vi "F8588A Digitizing Process.vi"(8 "error in":errorcluster, 11 "session in":variant) -> (0 "error out":errorcluster, 3 "aux data out":variant)   [LabVIEW 2020]
doc: "3458A digitizing lib: Main digitizing process. The VI is assynchronously executed once for each channel (all in parallel). It is started by calling 'Initiate Digitizing Process'. It then samples and sends the digitized data via queues to main process where the data are collected using 'Fetch Digitized Data'. Configuration of the execution is stored in 'session in' variable, execution control details are in 'session in->proc setup' cluster. Each instance of this VI has ID starting from 0 which identifies to which channel it belongs to."
uses:
  DMM/3458A Digitizer Session.ctl
  DMM/3458A Virtual Channel Config.ctl
  Counter/Counter Session.ctl
  Counter/Counter Type.ctl
  AWG/AWG Session.ctl
  AWG/AWG Type.ctl
  AWG/CMI Clock Divider v2/CMI ckd2 Session.ctl
  AWG/CMI Clock Divider v2/CMI ckd2 Source Mode.ctl
  AWG/CMI Sync V3/CMI Sync V3 session.ctl
  AWG/CMI Sync V3/Configure/CMI Sync V3 Reference Clock Source.ctl
  AWG/CMI Sync V3/Configure/CMI Sync V3 HV input Range.ctl
  AWG/CMI Sync V3/Configure/CMI Sync V3 Trigger Input Level.ctl
  AWG/CMI Sync V3/Configure/CMI Sync V3 Channel 1 Mode.ctl
  AWG/CMI Sync V3/Configure/CMI Sync V3 Channel Output Levels.ctl
  AWG/CMI Sync V3/Configure/CMI Sync V3 Channel 2 Mode.ctl
  AWG/CMI Sync V3/Configure/CMI Sync V3 Channel 3 Mode.ctl
  DMM/3458A Sync Mode.ctl
  DMM/3458A Idn Mode.ctl
  DMM/3458A Digitizing Low Levels/Configure/Sampling Mode.ctl
  DMM/3458A Digitizing Process Options.ctl
  DMM/3458A Data Packet.ctl
  DMM/3458A Aux Record Data.ctl
  DMM/3458A Digitizing Low Levels/Configure/Level Setup.ctl
  DMM/3458A Digitizing Low Levels/Configure/First Sample Trigger.ctl
  DMM/3458A Aperture Selection Mode.ctl
  DMM/3458A Multiplexing Config.ctl
  F8588A Low Pass Filter.ctl
  F8588A Phase Lock.ctl
  F8588A Coupling.ctl
  <vilib>/Utility/error.llb/Error Cluster From Error Code.vi
  <vilib>/ErrorRing/Error Ring.xnode
  DMM/3458A Virtual Digitizer.lvlib
  Counter/Counter.lvlib
  AWG/AWG.lvlib
  DMM/3458A Digitizing Low Levels/3458A Digitizing Low Levels.lvlib
  AWG/CMI Sync V3/CMI Sync Unit V3.lvlib
  AWG/AWG Clock Setup Mode.ctl
  DMM/3458A Sampling Rate.ctl
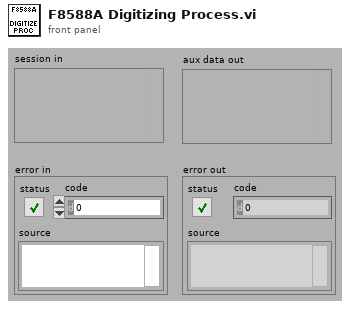
[diagram p1: front panel]
types:
  T1 = typedef "3458A Virtual Digitizer.lvlib/3458A Data Packet.ctl" = cluster{"data":i32[][], "offset [smpl]":i32, "count [smpl]":i32, "all done?":bool, "sampling?":bool, "queue buffer [%]":dbl, "valid?":bool, "overflow?":bool}
  T2 = typedef "3458A Virtual Digitizer.lvlib/3458A Digitizer Session.ctl" = cluster{"channels":T3[], "sync unit":T4, "awg unit":T6, "sync mode":T18, "streaming mode":bool, "idn mode":T19, "sampling mode":T20, "sample memory [B]":i32, "proc setup":T21, "sample size [B]":i32, "sample count":i32, "aux data":T23, "ranges [V]":dbl[], "aperture [s]":dbl, "LEVEL trigger":T24, "trigger mode":T25, "measure temp.?":bool, "disp mesages":string[], "shared bus?":bool, "disable display?":bool, "aper mode":T26, "aper rules":dbl[][], "multiplex":T27, "F8588 lpf":T28, "F8588 pll":T29, "F8588 couple":T30, "fs":T31}
  T3 = typedef "3458A Virtual Digitizer.lvlib/3458A Virtual Channel Config.ctl" = cluster{"VISA":refnum<visa-resource-name>, "Range [Vpk]":dbl, "btn clr":bool, "btn up":bool, "btn down":bool, "F8588":bool, "F8588 guard":bool}
  T4 = typedef "Counter.lvlib/Counter Session.ctl" = cluster{"VISA":refnum<visa-resource-name>, "type":T5}
  T5 = typedef "Counter.lvlib/Counter Type.ctl" = enum16{"Picotest U6200A", "dummy"}
  T6 = typedef "AWG.lvlib/AWG Session.ctl" = cluster{"type":T7, "VISA":refnum<visa-resource-name>, "enable 10MHz ref":bool, "cmi ckd2":T8, "cmi sync v3":T10}
  T7 = typedef "AWG.lvlib/AWG Type.ctl" = enum16{"Agilent 331xxA to 332xxA", "Agilent 335xxA to 336xxA", "Tektronix AFG3101C", "CMI Clock Divider v2", "CMI Sync Unit V3", "dummy"}
  T8 = typedef "AWG.lvlib/CMI ckd2 Session.ctl" = cluster{"VISA":refnum<visa-resource-name>, "clock source":T9, "manual ref clk":bool, "ref clock [Hz]":dbl}
  T9 = typedef "AWG.lvlib/CMI ckd2 Source Mode.ctl" = enum16{"Auto", "LF clock", "HF clock", "Internal"}
  T10 = typedef "AWG.lvlib/CMI Sync Unit V3.lvlib/CMI Sync V3 session.ctl" = cluster{"VISA":refnum<visa-resource-name>, "baud rate [bd/s]":i32, "source":T11, "hv range":T12, "fsrc is fixed":bool, "fsrc [Hz]":dbl, "freq integ [s]":dbl, "freq filter":i32, "trig level":T13, "chn1 mode":T14, "chn1 level":T15, "chn2 mode":T16, "chn2 level":T15, "chn2 div":i32, "chn3 mode":T17, "chn3 level":T15}
  T11 = typedef "AWG.lvlib/CMI Sync Unit V3.lvlib/CMI Sync V3 Reference Clock Source.ctl" = enum16{"Auto", "Internal", "Logic", "Sine", "HV"}
  T12 = typedef "AWG.lvlib/CMI Sync Unit V3.lvlib/CMI Sync V3 HV input Range.ctl" = enum16{"10V", "60V", "250V", "1kV"}
  T13 = typedef "AWG.lvlib/CMI Sync Unit V3.lvlib/CMI Sync V3 Trigger Input Level.ctl" = enum16{"LVCMOS 3V3", "TTL 5V"}
  T14 = typedef "AWG.lvlib/CMI Sync Unit V3.lvlib/CMI Sync V3 Channel 1 Mode.ctl" = enum16{"Source divider", "DDS absolute", "DDS ratio", "DDS ratio M/N"}
  T15 = typedef "AWG.lvlib/CMI Sync Unit V3.lvlib/CMI Sync V3 Channel Output Levels.ctl" = enum16{"Positive 3V3", "Negative 3V3", "Positive 5V", "Negative 5V"}
  T16 = typedef "AWG.lvlib/CMI Sync Unit V3.lvlib/CMI Sync V3 Channel 2 Mode.ctl" = enum16{"Source divider", "Chn 1 divide"}
  T17 = typedef "AWG.lvlib/CMI Sync Unit V3.lvlib/CMI Sync V3 Channel 3 Mode.ctl" = enum16{"Chn 1 Active", "Chn 2 Active", "Chn 1 Trigger", "Chn 2 Trigger", "Gate", "PPS", "10MHz"}
  T18 = typedef "3458A Virtual Digitizer.lvlib/3458A Sync Mode.ctl" = enum16{"MASTER-SLAVE, MASTER clocked by TIMER", "MASTER-SLAVE, MASTER clocked by AWG", "ALL clocked by AWG", "MASTER-SLAVE, ALL clocked by TIMER", "ALL clocked by AWG with DFLL"}
  T19 = typedef "3458A Virtual Digitizer.lvlib/3458A Idn Mode.ctl" = enum16{"Auto", "Sequential (chn A, chn B, ...)", "From calibration string"}
  T20 = typedef "3458A Virtual Digitizer.lvlib/3458A Digitizing Low Levels.lvlib/Sampling Mode.ctl" = enum16{"DCV", "DSDC", "DSAC"}
  T21 = typedef "3458A Virtual Digitizer.lvlib/3458A Digitizing Process Options.ctl" = cluster{"channel id":i32, "packet size [smpl]":i32, "current timeout [s]":dbl, "blk2blk timeout [s]":dbl, "event time":timestamp, "stop notifier":refnum<notifier>, "data queues":refnum<queue>[], "proc refs":refnum<vi>[], "bus semaphore":T22}
  T22 = typedef "Semaphore RefNum" = refnum<k1>
  T23 = typedef "3458A Virtual Digitizer.lvlib/3458A Aux Record Data.ctl" = cluster{"channel id":i32, "valid?":bool[], "gain [V]":dbl[], "timestamp [s]":dbl[], "Ts [s]":dbl, "abs timestamp":timestamp, "t [deg C]":dbl[], "multiplex timestamp [s]":dbl, "only multiplex?":bool, "multiplex smpl offset":i64, "overflow?":bool}
  T24 = typedef "3458A Virtual Digitizer.lvlib/3458A Digitizing Low Levels.lvlib/Level Setup.ctl" = cluster{"edge":enum16{"POS", "NEG"}, "level [V]":dbl, "coupling":enum16{"DC", "AC"}}
  T25 = typedef "3458A Virtual Digitizer.lvlib/3458A Digitizing Low Levels.lvlib/First Sample Trigger.ctl" = enum16{"AUTO", "EXT", "SYN", "SGL", "HOLD", "LEVEL"}
  T26 = typedef "3458A Virtual Digitizer.lvlib/3458A Aperture Selection Mode.ctl" = enum16{"Manual", "Maximum", "Table"}
  T27 = typedef "3458A Multiplexing Config.ctl" = cluster{"cycles":i32, "delay [s]":dbl, "enabled":bool, "overhead [s]":dbl, "tot smpls":i64, "sub-rec":i32, "overhead [%]":dbl, "emulated":bool}
  T28 = typedef "F8588A Low Pass Filter.ctl" = enum16{"Off", "100 kHz", "3 MHz"}
  T29 = typedef "F8588A Phase Lock.ctl" = enum16{"Off", "1 MHz", "10 MHz"}
  T30 = typedef "F8588A Coupling.ctl" = enum16{"AC, 1 MOhm", "AC, 10 MOhm", "DC, 1 MOhm", "DC, 10 MOhm", "DC, auto"}
  T31 = typedef "3458A Virtual Digitizer.lvlib/3458A Sampling Rate.ctl" = cluster{"freq mode":T32, "fs [Hz]":dbl, "fref [Hz]":dbl, "mul":dbl, "div":dbl}
  T32 = typedef "AWG.lvlib/AWG Clock Setup Mode.ctl" = enum16{"fs or Ts", "fs or Ts with fref", "fref/N", "fref*M/N", "fref*Ratio"}
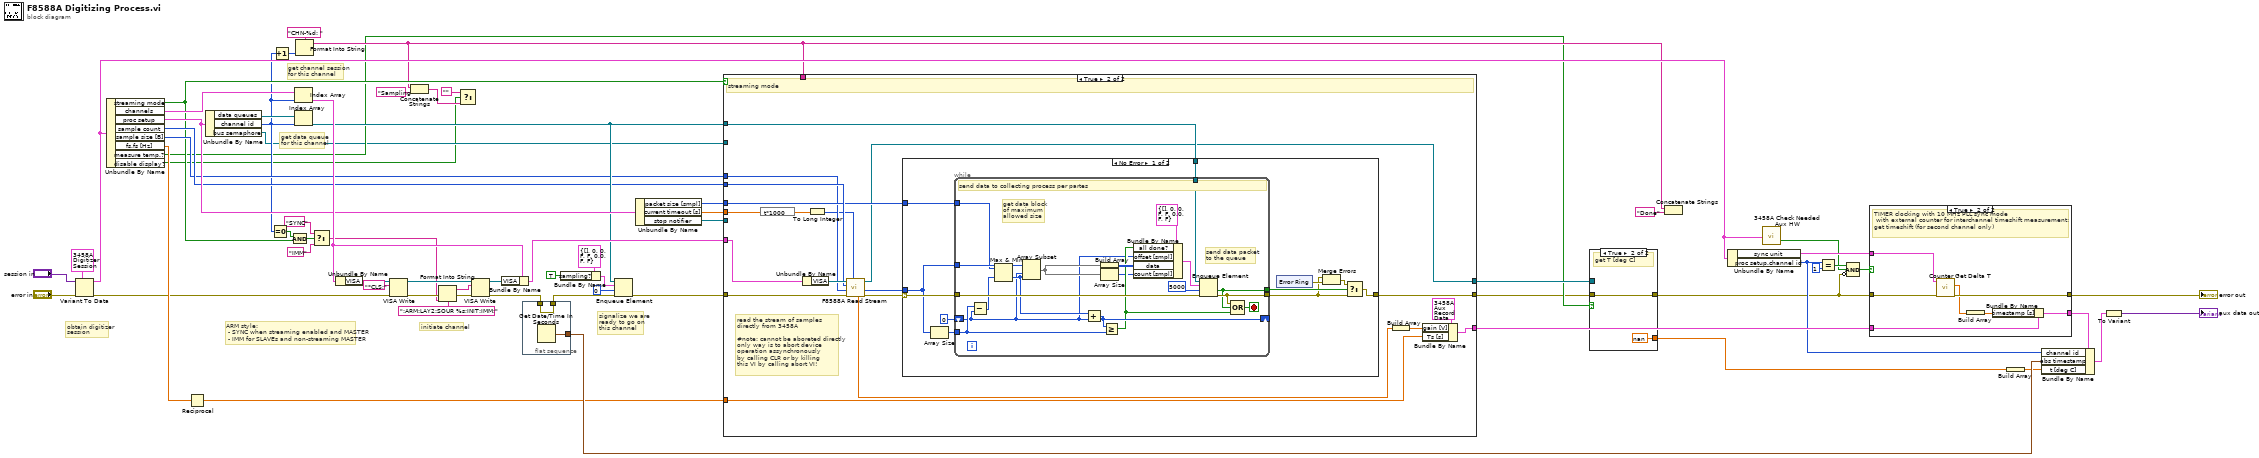
[diagram p0: block diagram]
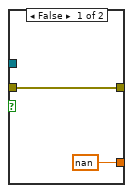
[diagram p2: hidden frame]
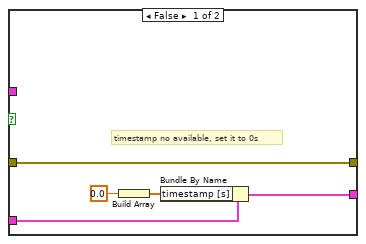
[diagram p3: hidden frame]
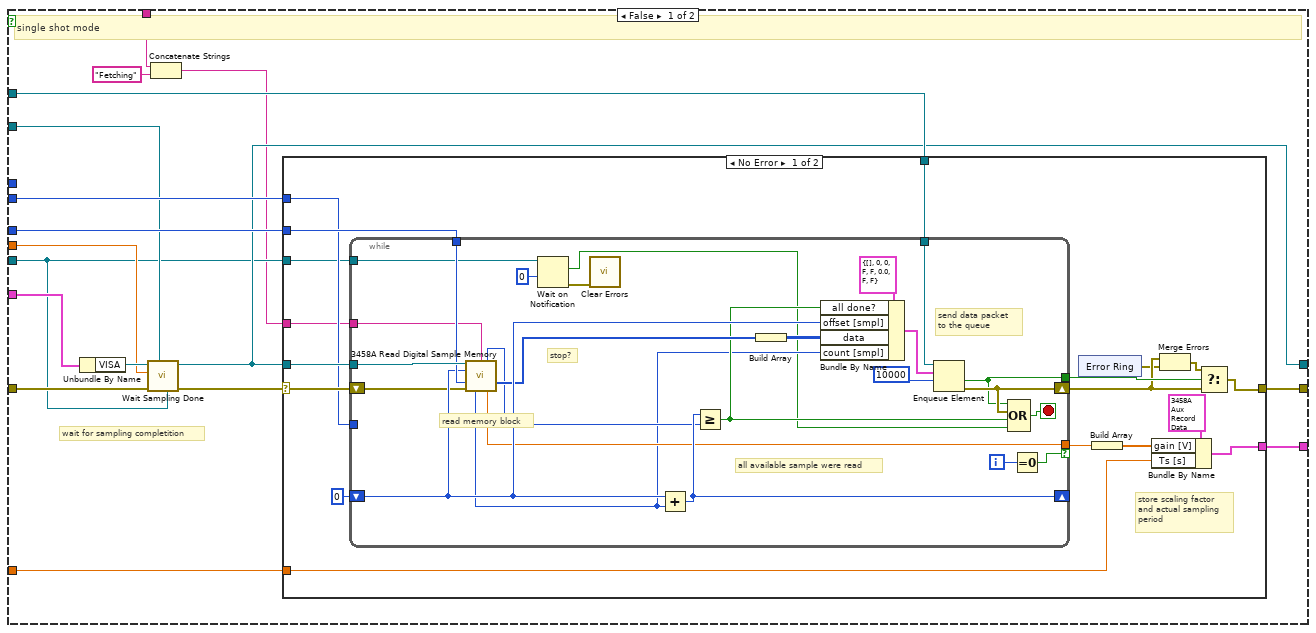
[diagram p4: hidden frame]
diagram:
  # "ARM style:\n - SYNC when streaming enabled and MASTER\n - IMM for SLAVEs and non-streaming MASTER"
  # "get channel session\nfor this channel"
  # "get data queue\nfor this channel"
  # "signalize we are\nready to go on \nthis channel"
  # "initiate channel"
  # "obtain digitizer\nsession"
  n1 = Variant To Data(error in="error in", type=T2 {"channels"=[], "sync unit"={"VISA"="", "type"=enum."Picotest U6200A"}, "awg unit"={"type"=enum."Agilent 331xxA to 332xxA", "VISA"="", "enable 10MHz ref"=FALSE, "cmi ckd2"={"VISA"="", "clock source"=enum."Auto", "manual ref clk"=FALSE, "ref clock [Hz]"=0.0}, "cmi sync v3"={"VISA"="", "baud rate [bd/s]"=115200, "source"=enum."Auto", "hv range"=enum."1kV", "fsrc is fixed"=FALSE, "fsrc [Hz]"=10000000.0, "freq integ [s]"=1.0, "freq filter"=5, "trig level"=enum."TTL 5V", "chn1 mode"=enum."Source divider", "chn1 level"=enum."Positive 5V", "chn2 mode"=enum."Source divider", "chn2 level"=enum."Positive 5V", "chn2 div"=1, "chn3 mode"=enum."Chn 1 Active", "chn3 level"=enum."Positive 5V"}}, "sync mode"=enum."MASTER-SLAVE, MASTER clocked by TIMER", "streaming mode"=FALSE, "idn mode"=enum."Auto", "sampling mode"=enum."DCV", "sample memory [B]"=0, "proc setup"={"channel id"=0, "packet size [smpl]"=0, "current timeout [s]"=0.0, "blk2blk timeout [s]"=0.0, "event time"=timestamp(0 s since 1904-01-01), "stop notifier"=refnum, "data queues"=[], "proc refs"=[], "bus semaphore"=refnum}, "sample size [B]"=0, "sample count"=0, "aux data"={"channel id"=0, "valid?"=[], "gain [V]"=[], "timestamp [s]"=[], "Ts [s]"=0.0, "abs timestamp"=timestamp(0 s since 1904-01-01), "t [deg C]"=[], "multiplex timestamp [s]"=-1.0, "only multiplex?"=FALSE, "multiplex smpl offset"=0, "overflow?"=FALSE}, "ranges [V]"=[], "aperture [s]"=0.0, "LEVEL trigger"={"edge"=enum."POS", "level [V]"=0.0, "coupling"=enum."DC"}, "trigger mode"=enum."AUTO", "measure temp.?"=FALSE, "disp mesages"=[], "shared bus?"=FALSE, "disable display?"=FALSE, "aper mode"=enum."Manual", "aper rules"=[], "multiplex"={"cycles"=0, "delay [s]"=0.0, "enabled"=FALSE, "overhead [s]"=1.0, "tot smpls"=0, "sub-rec"=0, "overhead [%]"=0.0, "emulated"=FALSE}, "F8588 lpf"=enum."Off", "F8588 pll"=enum."Off", "F8588 couple"=enum."DC, auto", "fs"={"freq mode"=enum."fs or Ts", "fs [Hz]"=0.0, "fref [Hz]"=0.0, "mul"=0.0, "div"=0.0}} ("digitizer session"), Variant="session in") -> (data=w45:T2, error out=w14:errorcluster)
  n2 = Unbundle By Name(w45) -> ("streaming mode"=w33:bool, "channels"=w65:T3[], "proc setup"=w57:T21, "sample count"=w52:i32, "sample size [B]"=w38:i32, "fs.fs [Hz]"=w35:dbl, "measure temp.?"=w22:bool, "disable display?"=w17:bool)
  n3 = Reciprocal(x=w35) -> (1/x=w1:dbl)
  n4 = Unbundle By Name(w57) -> ("data queues"=w64:refnum<queue>[], "channel id"=w28:i32, "bus semaphore"=w20:T22)
  n5 = Equal To 0?(x=w28) -> (x = 0?=w36:bool)
  n6 = Increment(x=w28) -> (x+1=w27:i32)
  n7 = Compound Arithmetic op=AND(w36, w33) -> (w37:bool)
  n8 = Index Array(array=w65, index=w28) -> (element=w63:T3)
  n9 = Index Array(array=w64, index=w28) -> (element=w53:refnum<queue>)
  n10 = Format Into String(format string="CHN-%d: ", w27) -> (resulting string=w23:string)  [unwired: 2 in, 1 out]
  n11 = Select(t="SYNC" ("string"), s=w37, f="IMM" ("string")) -> (s? t:f=w2:string)
  n12 = Unbundle By Name(w63) -> ("VISA"=w15:refnum<visa-resource-name>)
  n13 = VISA Write(VISA resource name=w15, write buffer="*CLS;", error in (no error)=w14) -> (VISA resource name out=w12:refnum<visa-resource-name>, error out=w9:errorcluster)  [unwired: 1 out]
  n14 = Concatenate Strings(w23, "Sampling" ("string")) -> (w18:string)
  n15 = Format Into String(format string=":ARM:LAY2:SOUR %s;INIT:IMM;" ("write buffer"), error in=w9, w2) -> (resulting string=w7:string, error out=w8:errorcluster)  [unwired: 1 in]
  n16 = Select(t="", s=w17, f=w18) -> ()  [unwired: 1 out]
  n17 = VISA Write(VISA resource name=w12, write buffer=w7, error in (no error)=w8) -> (VISA resource name out=w10:refnum<visa-resource-name>, error out=w11:errorcluster)  [unwired: 1 out]
  n18 = Bundle By Name(cluster=w63, "VISA"=w10) -> (w58:T3)
  n19 = flat-sequence {
    tunnel: w11 -> [w69]
    tunnel: [w69] -> w34
    tunnel: [w68] -> w31
    frame #0 {
      n20 = Get Date/Time In Seconds() -> (seconds since 1Jan1904=w68:timestamp)
    }
  }
  n21 = Bundle By Name(cluster=T1 {"data"=[], "offset [smpl]"=0, "count [smpl]"=0, "all done?"=FALSE, "sampling?"=FALSE, "queue buffer [%]"=0.0, "valid?"=FALSE, "overflow?"=FALSE} ("niScope packet"), "sampling?"=TRUE) -> (w60:T1)
  n22 = Enqueue Element(queue=w53, element=w60, timeout in ms (-1)=0, error in (no error)=w34) -> (error out=w39:errorcluster)  [unwired: 2 out]
  n23 = Unbundle By Name(w57) -> ("packet size [smpl]"=w54:i32, "current timeout [s]"=w56:dbl, "stop notifier"=w55:refnum<notifier>)
  n24 = case shown="True" w33 {
    tunnel: w39 -> [w78 w154]
    tunnel: w58 -> [w84 w153]
    tunnel: w56 -> [w85 w145]
    tunnel: w55 -> [w71 _]
    tunnel: w54 -> [w83 w143]
    tunnel: w53 -> [w82 w150]
    tunnel: w52 -> [w81 w151]
    tunnel: [w80 w142] -> w19
    tunnel: [w79 w148] -> w46
    tunnel: w38 -> [_ w141]
    tunnel: w1 -> [w77 w137]
    tunnel: [w73 w138] -> w32
    tunnel: w23 -> [w75 _]
    tunnel: w20 -> [w72 _]
    frame False {
      # "wait for sampling completition"
      # "single shot mode"
      n25 = Unbundle By Name(w84) -> ("VISA"=w86:refnum<visa-resource-name>)
      n26 = call "Wait Sampling Done.vi"("stop notifier ref (none)"=w71, "semaphore"=w72, "error in"=w78, "timeout [s] (5s)"=w85, "VISA resource in"=w86) -> ("error out"=w74:errorcluster, "VISA resource out"=w73:refnum<visa-resource-name>)  [unwired: 5 in]
      n27 = Concatenate Strings(w75, "Fetching" ("string")) -> (w70:string)
      n28 = case shown="No Error" w74 {
        selector: w74 -> [w103 w135]
        tunnel: w73 -> [w104 _]
        tunnel: w83 -> [w101 _]
        tunnel: w82 -> [w100 _]
        tunnel: w81 -> [w99 _]
        tunnel: [w93 w135] -> w80
        tunnel: [w96 _] -> w79
        tunnel: w77 -> [w89 _]
        tunnel: w70 -> [w88 _]
        tunnel: w71 -> [w87 _]
        frame No Error {
          # "store scaling factor\nand actual sampling\nperiod"
          n29 = while {
            tunnel: w104 -> [w131]
            shift-right: [w122] -> w91
            shift-left: w103 -> [w114]
            shift-right: [w126] -> _
            shift-left: 0 -> [w128]
            tunnel: w101 -> [w130]
            tunnel: w100 -> [w129]
            tunnel: w99 -> [_]
            tunnel: [w125] -> w97 if=w123
            tunnel: [w118] -> w94
            tunnel: w88 -> [w115]
            tunnel: w87 -> [w113]
            i -> [w124]
            stop <- w120 stop-if-true
            # "stop?"
            # "all available sample were read"
            # "read memory block"
            # "send data packet\nto the queue"
            n30 = call "3458A Read Digital Sample Memory.vi"("VISA session"=w131, "display string (none)"=w115, "First Read in Memory Location (0)"=w128, "max read [smpl]"=w130, "error in (no error)"=w114) -> ("total samples in memory?"=w117:i32, "waveform data int32"=w127:i32[], "read samples"=w116:i32, "scale factor"=w125:dbl)  [unwired: 4 in, 3 out]
            n31 = Wait on Notification(notifier=w113, timeout in ms (-1)=0) -> (notification=w110:bool, error out=w112:errorcluster)  [unwired: 2 in, 2 out]
            n32 = call <vilib>:"Clear Errors.vi"("error in (no error)"=w112) -> ()  [unwired: 5 in, 2 out]
            n33 = Add(x=w128, y=w116) -> (x+y=w126:i32)
            n34 = Greater Or Equal?(x=w126, y=w117) -> (x >= y?=w121:bool)
            n35 = Build Array(w127) -> (w119:i32[][])
            n36 = Bundle By Name(cluster=T1 {"data"=[], "offset [smpl]"=0, "count [smpl]"=0, "all done?"=FALSE, "sampling?"=FALSE, "queue buffer [%]"=0.0, "valid?"=FALSE, "overflow?"=FALSE} ("niScope packet"), "all done?"=w121, "offset [smpl]"=w128, "data"=w119, "count [smpl]"=w116) -> (w133:T1)
            n37 = Enqueue Element(queue=w129, element=w133, timeout in ms (-1)=10000) -> (timed out?=w118:bool, error out=w122:errorcluster)  [unwired: 1 in, 1 out]
            n38 = Compound Arithmetic op=OR(w118, w122, w121, w110) -> (w120:bool)
            n39 = Equal To 0?(x=w124) -> (x = 0?=w123:bool)
          }
          n40 = xnode "Error Ring"() -> ("error out"=w90:errorcluster)
          n41 = Build Array(w97) -> (w95:dbl[])
          n42 = Bundle By Name(cluster=T23 {"channel id"=0, "valid?"=[], "gain [V]"=[], "timestamp [s]"=[], "Ts [s]"=0.0, "abs timestamp"=timestamp(0 s since 1904-01-01), "t [deg C]"=[], "multiplex timestamp [s]"=0.0, "only multiplex?"=FALSE, "multiplex smpl offset"=0, "overflow?"=FALSE} ("aux data"), "gain [V]"=w95, "Ts [s]"=w89) -> (w96:T23)
          n43 = Merge Errors(w91, w90) -> (w92:errorcluster)
          n44 = Select(t=w92, s=w94, f=w91) -> (s? t:f=w93:errorcluster)
        }
        frame Error {
          # "timeout occured, do nothing"
        }
      }
    }
    frame True {
      # "read the stream of samples\ndirectly from 3458A\n\n#note: cannot be aboreted directly\nonly way is to abort device\noperation assynchronously\nby calling CLR or by killing\nthis VI by calling abort VI!"
      # "streaming mode"
      n45 = expression code="t*1000"(w145) -> (w144:dbl)
      n46 = Unbundle By Name(w153) -> ("VISA"=w152:refnum<visa-resource-name>)
      n47 = To Long Integer(number=w144) -> (32bit integer=w139:i32)
      n48 = call "F8588A Read Stream.vi"("read timeout [ms] (30000s)"=w139, "error in (no error)"=w154, "sample size [B]"=w141, "samples count"=w151, "VISA session"=w152) -> ("error out"=w140:errorcluster, "waveform data int32"=w136:i32[], "dup VISA session"=w138:refnum<visa-resource-name>, "scale factor"=w147:dbl)  [unwired: 1 in, 2 out]
      n49 = case shown="No Error" w140 {
        selector: w140 -> [w158 w190]
        tunnel: w150 -> [w165 _]
        tunnel: w136 -> [w155 _]
        tunnel: w143 -> [w163 _]
        tunnel: [w159 w190] -> w142
        frame No Error {
          n50 = Array Size(array=w155) -> (size(s)=w157:i32)
          n51 = while {
            tunnel: w158 -> [w186]
            tunnel: [w181] -> w156
            tunnel: w165 -> [w185]
            tunnel: w155 -> [w183]
            shift-right: [w182] -> _
            shift-left: 0 -> [w171]
            tunnel: w163 -> [w177]
            tunnel: w157 -> [w178]
            tunnel: [w179] -> w160
            stop <- w180 stop-if-true
            # "get data block\nof maximum\nallowed size"
            # "send data packet\nto the queue"
            # "send data to collecting process per partes"
            n52 = Subtract(x=w178, y=w171) -> (x-y=w176:i32)
            n53 = Max & Min(x=w177, y=w176) -> (min(x,y)=w175:i32)  [unwired: 1 out]
            n54 = Array Subset(array=w183, index=w171, length=w175) -> (w172:i32[])
            n55 = Add(x=w175, y=w171) -> (x+y=w182:i32)
            n56 = Build Array(w172) -> (w184:i32[][])
            n57 = Array Size(array=w172) -> (size(s)=w173:i32)
            n58 = Greater Or Equal?(x=w182, y=w178) -> (x >= y?=w174:bool)
            n59 = Bundle By Name(cluster=T1 {"data"=[], "offset [smpl]"=0, "count [smpl]"=0, "all done?"=FALSE, "sampling?"=FALSE, "queue buffer [%]"=0.0, "valid?"=FALSE, "overflow?"=FALSE} ("niScope packet"), "all done?"=w174, "offset [smpl]"=w171, "data"=w184, "count [smpl]"=w173) -> (w188:T1)
            n60 = Enqueue Element(queue=w185, element=w188, timeout in ms (-1)=5000, error in (no error)=w186) -> (timed out?=w179:bool, error out=w181:errorcluster)  [unwired: 1 out]
            n61 = Compound Arithmetic op=OR(w181, w179, w174) -> (w180:bool)
          }
          n62 = xnode "Error Ring"() -> ("error out"=w161:errorcluster)
          n63 = Merge Errors(w156, w161) -> (w162:errorcluster)
          n64 = Select(t=w162, s=w160, f=w156) -> (s? t:f=w159:errorcluster)
        }
        frame Error {
        }
      }
      n65 = Build Array(w147) -> (w149:dbl[])
      n66 = Bundle By Name(cluster=T23 {"channel id"=0, "valid?"=[], "gain [V]"=[], "timestamp [s]"=[], "Ts [s]"=0.0, "abs timestamp"=timestamp(0 s since 1904-01-01), "t [deg C]"=[], "multiplex timestamp [s]"=0.0, "only multiplex?"=FALSE, "multiplex smpl offset"=0, "overflow?"=FALSE} ("aux data"), "gain [V]"=w149, "Ts [s]"=w137) -> (w148:T23)
    }
  }
  n67 = case shown="True" w22 {
    tunnel: w19 -> [w192 w194]
    tunnel: [w192 w194] -> w3
    tunnel: w32 -> [_ _]
    tunnel: [nan nan] -> w30
    frame False {
    }
    frame True {
      # "get T [deg C]"
    }
  }
  n68 = Concatenate Strings(w23, "Done" ("string")) -> ()  [unwired: 1 out]
  n69 = Unbundle By Name(w45) -> ("sync unit"=w49:T4, "proc setup.channel id"=w40:i32)
  n70 = call "3458A Check Needed Aux HW.vi"("digitizer session"=w45) -> ("uses counter for delta T sync?"=w44:bool)  [unwired: 13 in, 5 out]
  n71 = Equal?(x=w40, y=1) -> (x = y?=w47:bool)
  n72 = Compound Arithmetic op=AND(w47, w44, invert w3) -> (w50:bool)
  n73 = case shown="True" w50 {
    tunnel: w3 -> [w199 w203]
    tunnel: w49 -> [_ w201]
    tunnel: w46 -> [w197 w206]
    tunnel: [w199 w202] -> w21
    tunnel: [w198 w205] -> w41
    frame False {
      # "timestamp no available, set it to 0s"
      n74 = Build Array(0.0 ("time stamp [s]")) -> (w196:dbl[])
      n75 = Bundle By Name(cluster=w197, "timestamp [s]"=w196) -> (w198:T23)
    }
    frame True {
      # "TIMER clocking with 10 MHz PLL sync mode\n with external counter for interchannel timeshift measurement:\nget timeshift (for second channel only)"
      n76 = call "Counter Get Delta T.vi"("error in"=w203, "counter session in"=w201) -> ("error out"=w202:errorcluster, "delta t [s]"=w200:dbl)  [unwired: 7 in, 1 out]
      n77 = Build Array(w200) -> (w204:dbl[])
      n78 = Bundle By Name(cluster=w206, "timestamp [s]"=w204) -> (w205:T23)
    }
  }
  "error out" <- w21
  n79 = Build Array(w30) -> (w29:dbl[])
  n80 = Bundle By Name(cluster=w41, "channel id"=w40, "abs timestamp"=w31, "t [deg C]"=w29) -> (w42:T23)
  n81 = To Variant(anything=w42) -> (Variant=→"aux data out":variant)
